vi "Sort Panels.vi"(8 "error in (no error)":errorcluster, 11 "ArrayManager in":refnum<class "ArrayManager.lvclass">) -> (0 "error out":errorcluster, 2 "Sorted ArrayPanels":refnum<class "ArrayPanel.lvclass">[](array[class]), 3 "ArrayManager out":refnum<class "ArrayManager.lvclass">)   [LabVIEW 2020, in "OOPanel.lvlib" / "ArrayManager.lvclass"]
uses:
  ArrayManager.lvclass
  Sort VI Type.ctl
  Panel/Panel.lvclass
  ArrayPanel/ArrayPanel.lvclass
panel:
  in  "Sort VI":T1
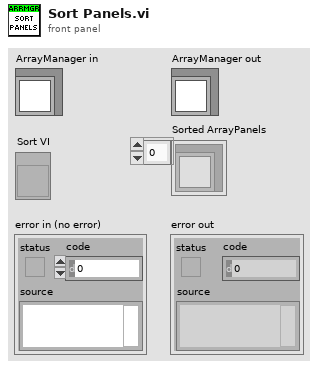
[diagram p1: front panel]
types:
  T1 = typedef "OOPanel.lvlib/ArrayManager.lvclass/Sort VI Type.ctl" = refnum<vi>
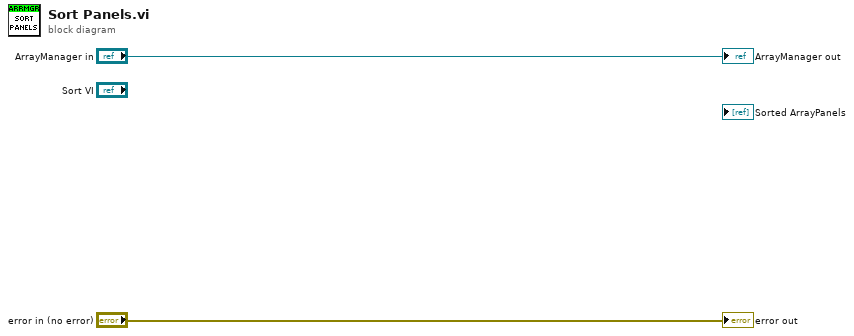
[diagram p0: block diagram]
diagram:
  "error out" <- "error in (no error)"
  "ArrayManager out" <- "ArrayManager in"
